vi "Develop Tools - ScratchPopulate.vi"() -> ()   [LabVIEW 2011]
panel:
  in  "9_2":T1 {"HSlide" scale=0.0..10.0; "VSlide" scale=0.0..10.0}
  in  "8_2":T1 {"HSlide" scale=0.0..10.0; "VSlide" scale=0.0..10.0}
  in  "7_2":T1 {"HSlide" scale=0.0..10.0; "VSlide" scale=0.0..10.0}
  in  "6_2":T1 {"HSlide" scale=0.0..10.0; "VSlide" scale=0.0..10.0}
  in  "5_2":T1 {"HSlide" scale=0.0..10.0; "VSlide" scale=0.0..10.0}
  in  "4_2":T1 {"HSlide" scale=0.0..10.0; "VSlide" scale=0.0..10.0}
  in  "3_2":T1 {"HSlide" scale=0.0..10.0; "VSlide" scale=0.0..10.0}
  in  "2_2":T1 {"HSlide" scale=0.0..10.0; "VSlide" scale=0.0..10.0}
  in  "1_2":T1 {"HSlide" scale=0.0..10.0; "VSlide" scale=0.0..10.0}
  in  "0_2":T1 {"HSlide" scale=0.0..10.0; "VSlide" scale=0.0..10.0}
  in  "9_1":T1 {"HSlide" scale=0.0..10.0; "VSlide" scale=0.0..10.0}
  in  "8_1":T1 {"HSlide" scale=0.0..10.0; "VSlide" scale=0.0..10.0}
  in  "7_1":T1 {"HSlide" scale=0.0..10.0; "VSlide" scale=0.0..10.0}
  in  "6_1":T1 {"HSlide" scale=0.0..10.0; "VSlide" scale=0.0..10.0}
  in  "5_1":T1 {"HSlide" scale=0.0..10.0; "VSlide" scale=0.0..10.0}
  in  "4_1":T1 {"HSlide" scale=0.0..10.0; "VSlide" scale=0.0..10.0}
  in  "3_1":T1 {"HSlide" scale=0.0..10.0; "VSlide" scale=0.0..10.0}
  in  "2_1":T1 {"HSlide" scale=0.0..10.0; "VSlide" scale=0.0..10.0}
  in  "1_1":T1 {"HSlide" scale=0.0..10.0; "VSlide" scale=0.0..10.0}
  in  "0_1":T1 {"HSlide" scale=0.0..10.0; "VSlide" scale=0.0..10.0}
  in  "9_0":T1 {"HSlide" scale=0.0..10.0; "VSlide" scale=0.0..10.0}
  in  "8_0":T1 {"HSlide" scale=0.0..10.0; "VSlide" scale=0.0..10.0}
  in  "7_0":T1 {"HSlide" scale=0.0..10.0; "VSlide" scale=0.0..10.0}
  in  "6_0":T1 {"HSlide" scale=0.0..10.0; "VSlide" scale=0.0..10.0}
  in  "5_0":T1 {"HSlide" scale=0.0..10.0; "VSlide" scale=0.0..10.0}
  in  "4_0":T1 {"HSlide" scale=0.0..10.0; "VSlide" scale=0.0..10.0}
  in  "3_0":T1 {"HSlide" scale=0.0..10.0; "VSlide" scale=0.0..10.0}
  in  "2_0":T1 {"HSlide" scale=0.0..10.0; "VSlide" scale=0.0..10.0}
  in  "1_0":T1 {"HSlide" scale=0.0..10.0; "VSlide" scale=0.0..10.0}
  in  "0_0":T1 {"HSlide" scale=0.0..10.0; "VSlide" scale=0.0..10.0}
types:
  T1 = cluster{"Box":dbl[unit], "Spin":dbl[unit], "VSlide":dbl[unit], "HSlide":dbl[unit], "Push Button":bool, "HRocker":bool, "VRocker":bool, "HToggle":bool, "VToggle":bool, "HSlideSW":bool, "VSlideSW":bool, "System":bool, "Square Push Button":bool, "Round Push Button":bool, "VSlideSW2":bool, "Square Push Btn2":bool, "Round Push Btn2":bool, "HSlideSW2":bool, "Round LED":bool, "Square LED":bool}
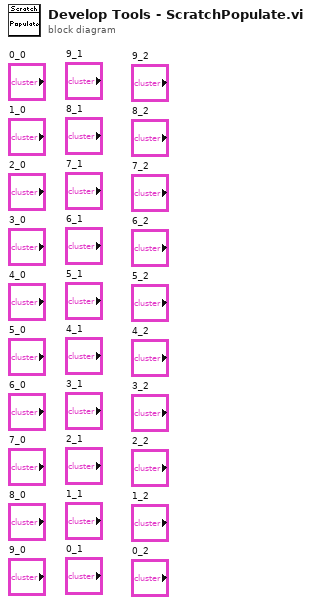
[diagram p0: block diagram]
diagram:
